vi "Open Dynamic VI.vi"(8 "error in (no error)":errorcluster, 11 "vi path":path) -> (0 "error out":errorcluster, 3 "VI out":refnum<vi>)   [LabVIEW 2020]
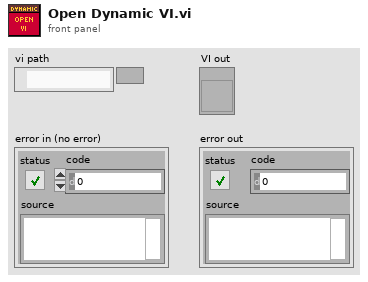
[diagram p1: front panel]
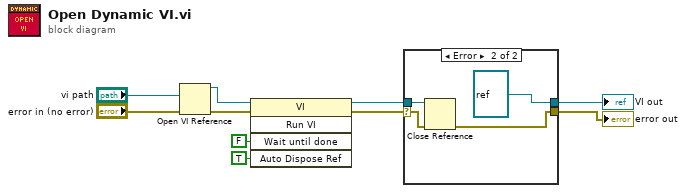
[diagram p0: block diagram]
diagram:
  n1 = Open VI Reference(vi path="vi path", error in (no error)="error in (no error)") -> (vi reference=w7:refnum<vi>, error out=w5:errorcluster)  [unwired: 4 in]
  n2 = invoke class="VI" method="Run VI"(reference=w7, error in=w5, "Wait until done"=FALSE ("Wait Until Done"), "Auto Dispose Ref"=TRUE ("Auto Dispose Reference")) -> (reference out=w3:refnum<vi>, error out=w4:errorcluster)  [unwired: 1 in, 3 out]
  n3 = case shown="Error" w4 {
    selector: w4 -> [w11 w15]
    tunnel: w3 -> [w12 w16]
    tunnel: [w12 refnum<vi> refnum] -> w2
    tunnel: [w11 w14] -> w1
    frame No Error {
    }
    frame Error {
      n4 = Close Reference(reference=w16, error in (no error)=w15) -> (error out=w14:errorcluster)
    }
  }
  "VI out" <- w2
  "error out" <- w1
